vi "Wire Input Param.vi"(4 "Default C++ Value":string, 6 "ConPane Terminal Index":u32, 7 "CallLibrary Terminal Index":i32, 9 "CalllLibrary Ref":refnum<vi>, 10 "VI Ref":refnum<vi>, 11 "Abstract Param Writer in":refnum<class "Abstract Param Writer.lvclass">) -> (3 "Abstract Param Writer out":refnum<class "Abstract Param Writer.lvclass">)   [LabVIEW 2013, in "Abstract Param Writer.lvclass"]
doc: "Copyright (c) 2016 Sze Howe Koh\n\nThis Source Code Form is subject to the terms of the Mozilla Public License, v. 2.0. If a copy of the MPL was not distributed with this file, You can obtain one at http://mozilla.org/MPL/2.0/."
uses:
  Abstract Param Writer.lvclass
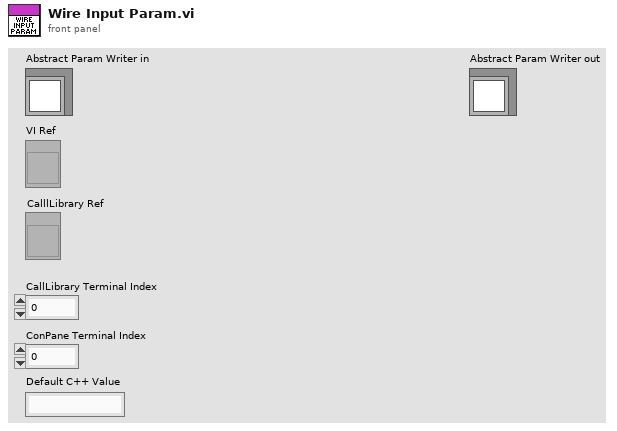
[diagram p1: front panel]
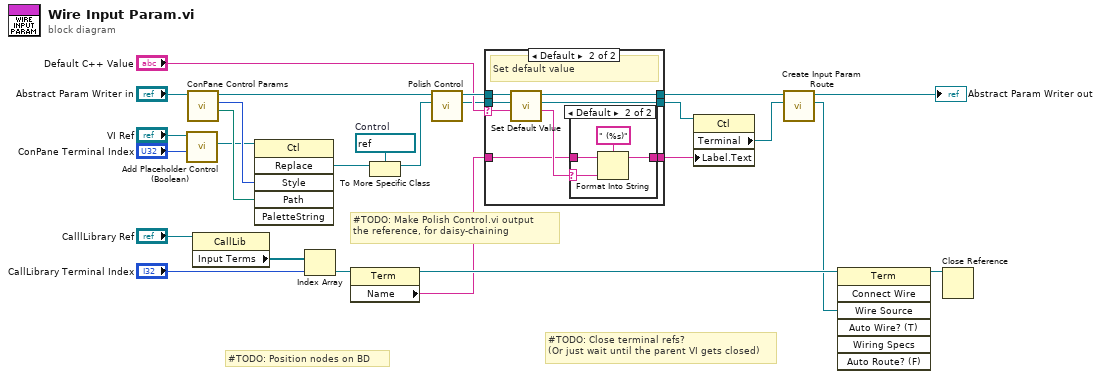
[diagram p0: block diagram]
diagram:
  w16 = refnum<vi> refnum  # Control
  # "#TODO: Make Polish Control.vi output\nthe reference, for daisy-chaining"
  # "#TODO: Close terminal refs?\n(Or just wait until the parent VI gets closed)"
  # "#TODO: Position nodes on BD"
  n1 = call "Add Placeholder Control (Boolean).vi"("ConPane Terminal Index"="ConPane Terminal Index", "VI Ref"="VI Ref") -> ("Control Ref"=w18:refnum<vi>)  [unwired: 9 in]
  n2 = call-dynamic "ConPane Control Params.vi"("Abstract Param Writer in"="Abstract Param Writer in") -> ("Path"=w19:path, "Style"=w20:i32, "Abstract Param Writer out"=w9:refnum<class "Abstract Param Writer.lvclass">)  [unwired: 8 in]
  n3 = property class="CallLib"(reference="CalllLibrary Ref") -> ("Input Terms"=w24:refnum<vi>[])  [unwired: 1 in, 2 out]
  n4 = invoke class="Ctl" method="Replace"(reference=w18, "Style"=w20, "Path"=w19) -> ("Replace"=w17:refnum<vi>)  [unwired: 3 in, 5 out]
  n5 = Index Array(array=w24, index="CallLibrary Terminal Index") -> (element=w23:refnum<vi>)
  n6 = property class="Term"(reference=w23) -> (reference out=w15:refnum<vi>, "Name"=w5:string)  [unwired: 1 in, 1 out]
  n7 = To More Specific Class(target class=w16, reference=w17) -> (specific class reference=w1:refnum<vi>)  [unwired: 1 in, 1 out]
  n8 = call-dynamic "Polish Control.vi"("Control Ref"=w1, "Abstract Param Writer in"=w9) -> ("Abstract Param Writer out"=w8:refnum<class "Abstract Param Writer.lvclass">)  [unwired: 9 in]
  n9 = case shown="Default" "Default C++ Value" {
    selector: "Default C++ Value" -> [_ w33]
    tunnel: w8 -> [w28 w36]
    tunnel: [w28 w35] -> w7
    tunnel: w1 -> [w26 w34]
    tunnel: w5 -> [w27 w31]
    tunnel: [w27 w30] -> w2
    tunnel: [w26 w29] -> w4
    frame "" {
      # "No default specified"
    }
    frame Default {
      # "Set default value"
      n10 = call-dynamic "Set Default Value.vi"("Default C++ Value"=w33, "Control Ref"=w34, "Abstract Param Writer in"=w36) -> ("LabVIEW Default String"=w32:string, "Control Ref Dup"=w29:refnum<vi>, "Abstract Param Writer out"=w35:refnum<class "Abstract Param Writer.lvclass">)  [unwired: 6 in]
      n11 = case shown="Default" w32 {
        selector: w32 -> [_ w40]
        tunnel: w31 -> [w37 w41]
        tunnel: [w37 w38] -> w30
        frame "" {
        }
        frame Default {
          n12 = Format Into String(format string=" (%s)", initial string=w41, w40) -> (resulting string=w38:string)  [unwired: 1 in, 1 out]
        }
      }
    }
  }
  n13 = property class="Ctl"(reference=w4, "Label.Text"=w2) -> ("Terminal"=w3:refnum<vi>)  [unwired: 1 in, 2 out]
  n14 = call-dynamic "Create Input Param Route.vi"("Control Terminal"=w3, "Abstract Param Writer in"=w7) -> ("CLFN Terminal Source"=w12:refnum<vi>, "Abstract Param Writer out"=→"Abstract Param Writer out":refnum<class "Abstract Param Writer.lvclass">)  [unwired: 8 in]
  n15 = invoke class="Term" method="Connect Wire"(reference=w15, "Wire Source"=w12) -> (reference out=w14:refnum<vi>)  [unwired: 5 in, 6 out]
  n16 = Close Reference(reference=w14) -> ()  [unwired: 1 in, 1 out]
